vi "Process.vi"(8 "error in":errorcluster, 11 "Instrument UI.FrameworkTemplate":refnum<class "Instrument UI.Temperhum.lvclass">) -> (0 "error out":errorcluster, 3 "Instrument UI.FrameworkTemplate out":refnum<class "Instrument UI.Temperhum.lvclass">)   [LabVIEW 2019, in "Instrument UI.Temperhum.lvclass"]
doc: "---------------------------------------------------------------\nJKI State Machine Objects™\nhttp://jki.net/state-machine-objects/\nCopyright (C) 2005-2015, JKI <info@jki.net>\nALL RIGHTS RESERVEDJKI State Machine Objects (SMO) 1.0.0.5\nJKI - JKI\nCopyright (c) 2016, JKI"
uses:
  Instrument UI.Temperhum.lvclass
  C:/Program Files (x86)/National Instruments/LabVIEW 2019/vi.lib/JKI/JKI SMO/SMO/SMO.lvclass
  C:/Program Files (x86)/National Instruments/LabVIEW 2019/user.lib/LevyLab/Instrument Framework/SMOs/Instrument UI/Instrument UI.lvclass
  C:/Program Files (x86)/National Instruments/LabVIEW 2019/vi.lib/JKI/JKI SMO/SMO.UI/SMO.UI.lvclass
  <vilib>/JKI/JKI SMO/SMO/Typedefs/Parent Call--Enum.ctl
  Instrument.Temperhum/Typedefs/Instrument.Temperhum.getAll--Cluster.ctl
  Instrument.Temperhum/Instrument.Temperhum.lvclass
  C:/Program Files (x86)/National Instruments/LabVIEW 2019/user.lib/LevyLab/Instrument Framework/SMOs/Instrument/Instrument.lvclass
  Instrument UI.Temperhum.UI--Cluster.ctl
  Instrument.Temperhum/Typedefs/Instrument.Temperhum.Configuration--Cluster.ctl
  <userlib>/LevyLab/Instrument Framework/SMOs/Configuration/Configuration.lvclass
  <userlib>/LevyLab/Instrument Framework/SMOs/Instrument UI/Instrument UI.lvclass/Instrument UI.ctl
  Instrument.Temperhum/Instrument.Temperhum.lvclass/Instrument.Temperhum.ctl
  <vilib>/JKI/JKI SMO/SMO/SMO.lvclass/SMO.ctl
  <userlib>/LevyLab/Instrument Framework/SMOs/Instrument/Instrument.lvclass/Instrument.ctl
  614f1787-3484-4d72-b522-1f8c221dac07.vi
  064e3a37-d4cf-416d-9c97-81a00de9d50c.vi
  <vilib>/JKI/JKI SMO/SMO/Private/ReftoDVR--SMO.vi
  614f1787-3484-4d72-b522-1f8c221dac07.vi/0804abc2-d62d-4fc2-83e4-fbfa93b6771f.vi
  064e3a37-d4cf-416d-9c97-81a00de9d50c.vi/63d05343-f2e5-4332-a01c-367bfd4ece1f.vi
  614f1787-3484-4d72-b522-1f8c221dac07.vi/0804abc2-d62d-4fc2-83e4-fbfa93b6771f.vi/49ab1656-e913-41b8-8f65-7ccb5614f4ae.vi
  <userlib>/LevyLab/Instrument Framework/SMOs/Instrument/API/Send and Receive.vi
  <userlib>/LevyLab/Instrument Framework/SMOs/Instrument/API/Read SMO Address.vi
  064e3a37-d4cf-416d-9c97-81a00de9d50c.vi/63d05343-f2e5-4332-a01c-367bfd4ece1f.vi/e8b685cb-2eaa-4147-917d-8853431d5f1e.vi
  614f1787-3484-4d72-b522-1f8c221dac07.vi/0804abc2-d62d-4fc2-83e4-fbfa93b6771f.vi/49ab1656-e913-41b8-8f65-7ccb5614f4ae.vi/5f920abd-0665-4854-95b0-22af96bc7ab8.vi
  614f1787-3484-4d72-b522-1f8c221dac07.vi/0804abc2-d62d-4fc2-83e4-fbfa93b6771f.vi/49ab1656-e913-41b8-8f65-7ccb5614f4ae.vi/ccf45d59-ecb4-4ff7-9932-c5d6b9216eb0.vi
  064e3a37-d4cf-416d-9c97-81a00de9d50c.vi/63d05343-f2e5-4332-a01c-367bfd4ece1f.vi/e8b685cb-2eaa-4147-917d-8853431d5f1e.vi/8176c5a5-7aad-4107-91e7-ec137d50c96d.vi
  064e3a37-d4cf-416d-9c97-81a00de9d50c.vi/63d05343-f2e5-4332-a01c-367bfd4ece1f.vi/e8b685cb-2eaa-4147-917d-8853431d5f1e.vi/514d73de-289c-4ab7-be0e-afcbb581ae6d.vi
  <userlib>/LevyLab/Instrument Framework/SMOs/Instrument/API/Enum to String.vi
  <userlib>/LevyLab/Instrument Framework/SMOs/RemoteControl/API/Send and Receive.vi
  <vilib>/Utility/Data Type/Get Type Information.vi
  <vilib>/JDP Science/JSONtext/JSON text to Variant.vi
  <userlib>/LevyLab/Instrument Framework/SMOs/Instrument/Instrument.lvclass
  <vilib>/JDP Science/JSONtext/LVClass Serializer/JSONtext LVClass Serializer.lvclass
  <userlib>/LevyLab/Instrument Framework/SMOs/Instrument UI/Instrument UI.lvclass
  <vilib>/JKI/JKI SMO/SMO/SMO.lvclass
  <vilib>/JKI/JKI SMO/SMO.UI/SMO.UI.lvclass
  <userlib>/LevyLab/LV-Data/LV-Data.PG/LV-Data.PGSQL.lvclass
panel:
  out "PGSQL":string
  out "TH Graph":cluster{timestamp[], dbl[]}[](graph)
  out "Hardware Type":string
  out "Numeric":u32
  in  "STOP":bool
  out "Humidity (%RH)":dbl
  out "Temperature (K)":dbl
  # "SMO UI Template"
  # "For instructions on how to use the JKI State Machine Objects, examples and video tutorials, visit:\nhttp://jki.net/state-machine-objects/\n\nJKI State Machine Objects™\nhttp://jki.net/state-machine-objects/\nCopyright (C) 2005-2015, JKI <info@jki.net>\nALL RIGHTS RESERVED"
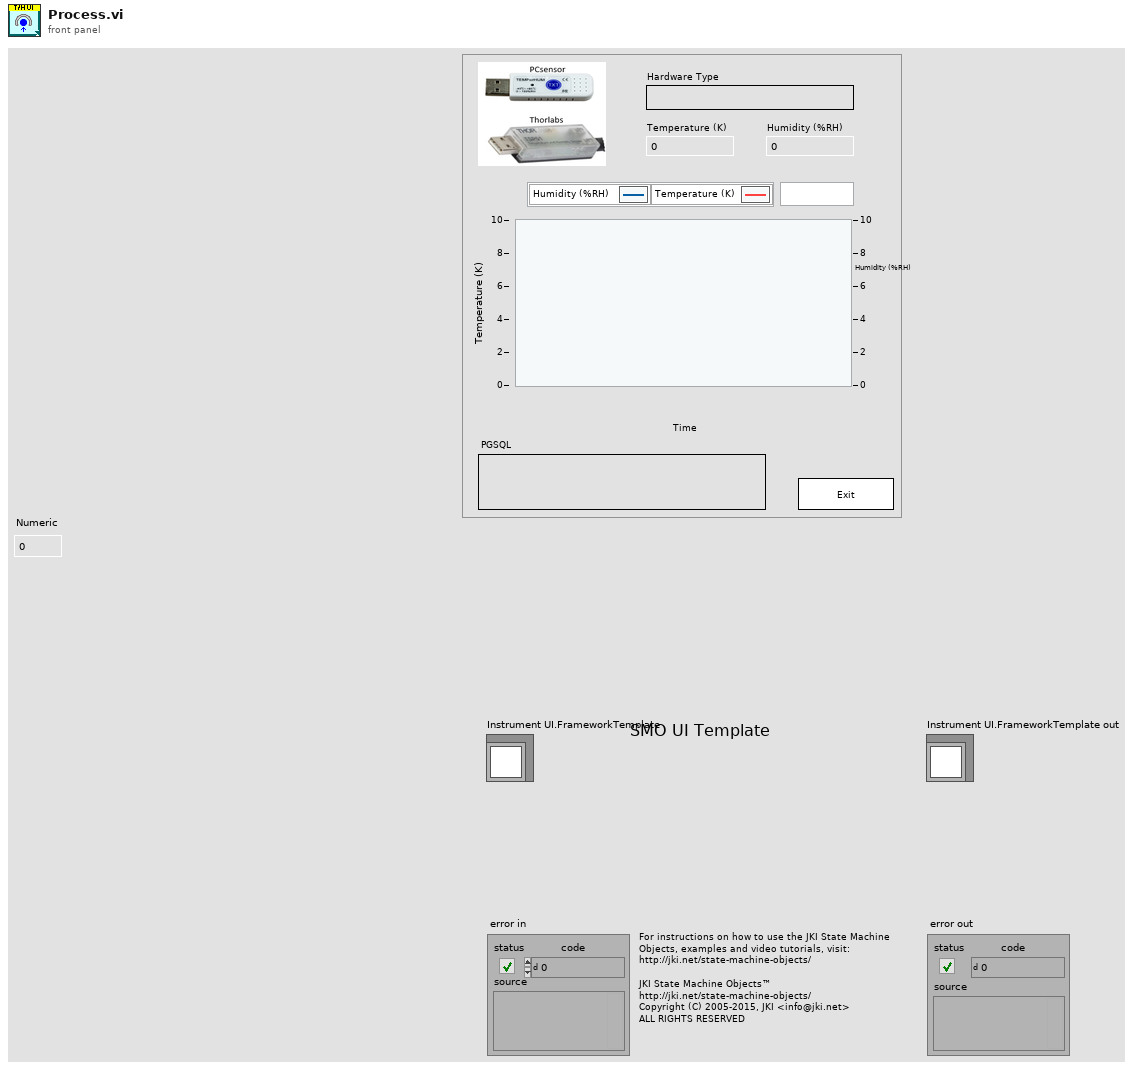
[diagram p1: front panel]
types:
  T1 = typedef "SMO.lvclass/Parent Call--Enum.ctl" = enum16{"Allows parent to run", "Does not request parent to run"}
  T2 = enum32{"invalid app kind", "Development System", "Run Time System", "Student Edition", "Embedded LabVIEW", "Evaluation", "Custom"}
  T3 = enum32{"Invalid", "Standard", "Closed", "Hidden", "Minimized", "Maximized"}
  T4 = typedef "Instrument.Temperhum.lvclass/Instrument.Temperhum.getAll--Cluster.ctl" = cluster{"Temperature (K)":dbl, "Humidity (%RH)":dbl}
  T5 = typedef "Instrument.Temperhum.lvclass/Instrument.Temperhum.Configuration--Cluster.ctl" = cluster{"Example Setting 1":dbl, "Example Setting 2":dbl, "Logpath":string}
  T6 = typedef "Instrument UI.Temperhum.lvclass/Instrument UI.Temperhum.UI--Cluster.ctl" = cluster{"Parameter":dbl, "Parameter 2":string}
  T7 = cluster{"Core":cluster{"Current VI Reference":refnum<vi>, "Close Panel on Exit?":bool, "error":errorcluster}, "Instrument UI":refnum<class "Instrument UI.Temperhum.lvclass">, "Instrument":refnum<class "Instrument.Temperhum.lvclass">, "Configuration":refnum<class "Configuration.lvclass">, "Config Cluster":T5, "getAll":T4, "UI Cluster":T6}
  T8 = typedef "Instrument.Temperhum.lvclass/PublicEvents--Instrument.Temperhum.Get PGSQL Info.ctl" = string
  T9 = cluster{"Current VI Reference":refnum<vi>, "Close Panel on Exit?":bool, "error":errorcluster}
  T10 = typedef "SMO.lvclass/Protected Events.ctl" = cluster{"StopProcesses":refnum<user-event>, "AbortProcesses":refnum<user-event>, "Config Changed":refnum<user-event>, "Dependency":refnum<user-event>}
  T11 = typedef "Instrument.lvclass/PublicEvents--Cluster.ctl" = cluster{"MessageFromProcess":refnum<user-event>}
  T12 = typedef "Instrument.Temperhum.lvclass/PublicEvents--Cluster.ctl" = cluster{"Get PGSQL Info":refnum<user-event>}
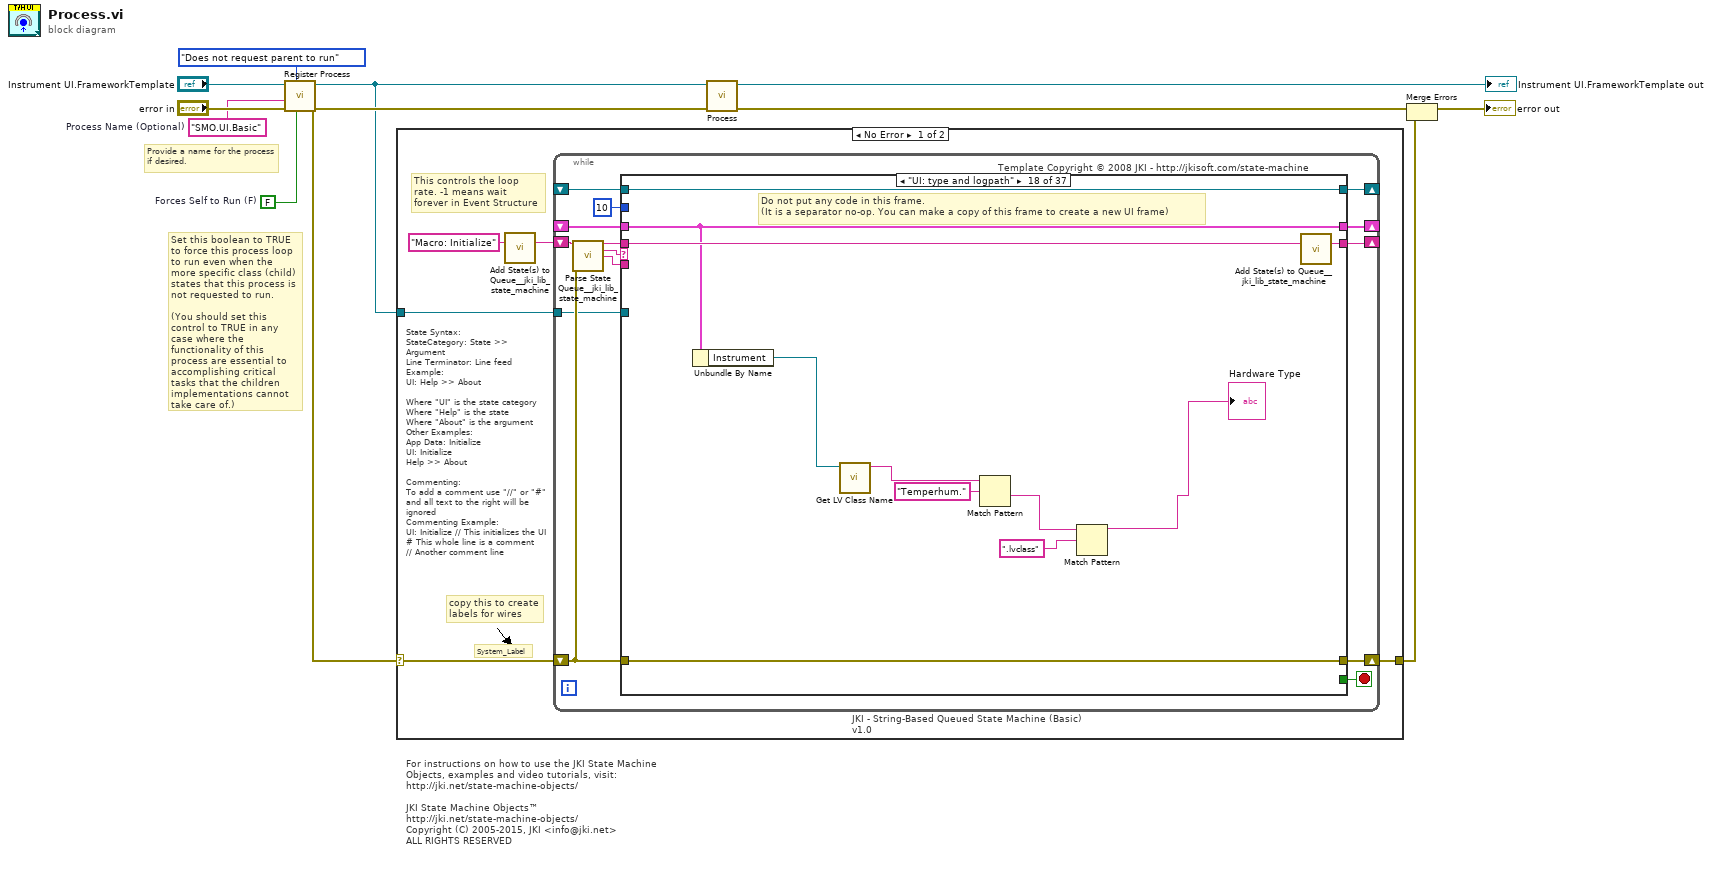
[diagram p0: block diagram]
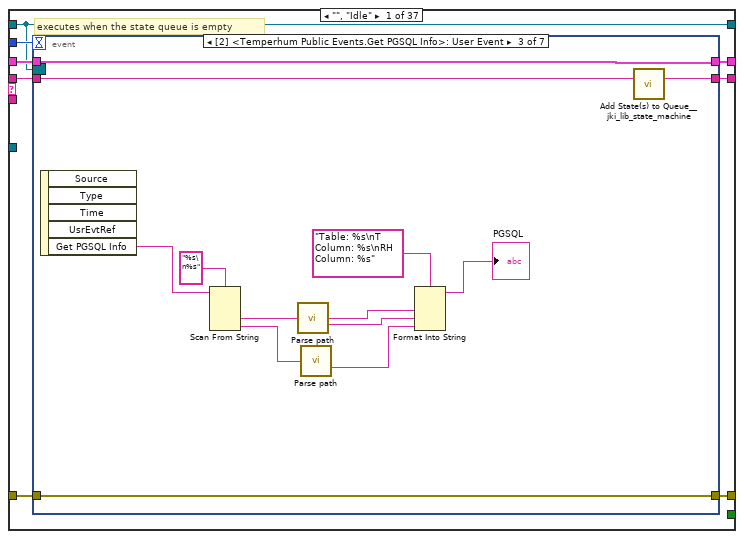
[diagram p2: hidden frame]
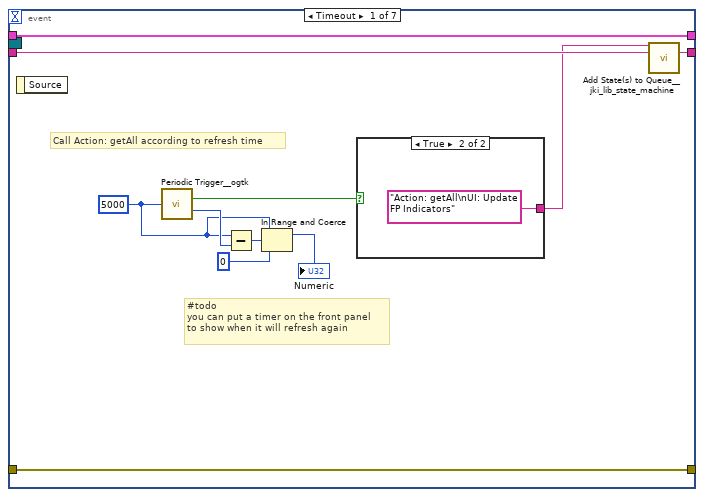
[diagram p3: hidden frame]
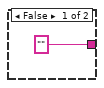
[diagram p4: hidden frame]
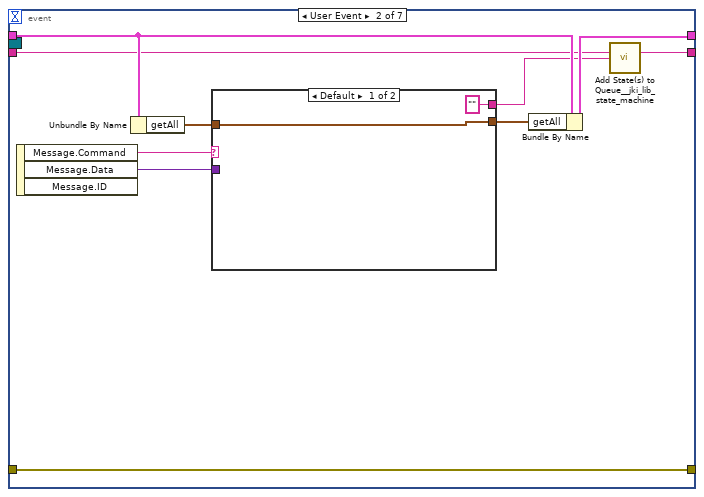
[diagram p5: hidden frame]
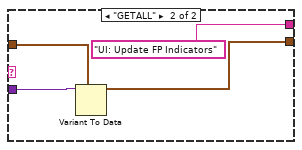
[diagram p6: hidden frame]
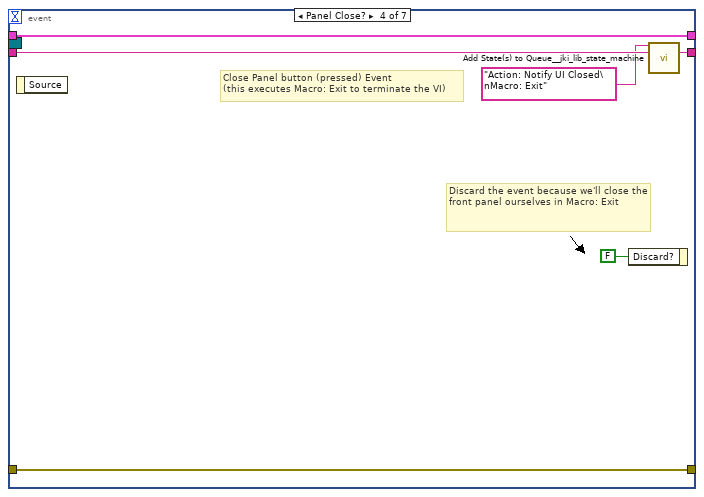
[diagram p7: hidden frame]
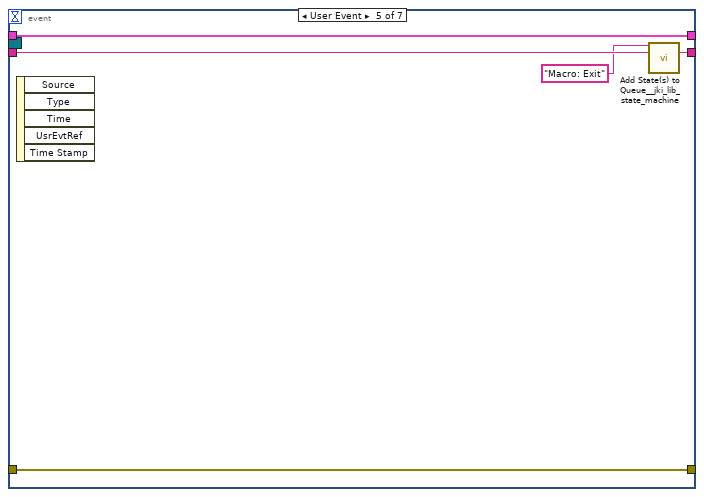
[diagram p8: hidden frame]
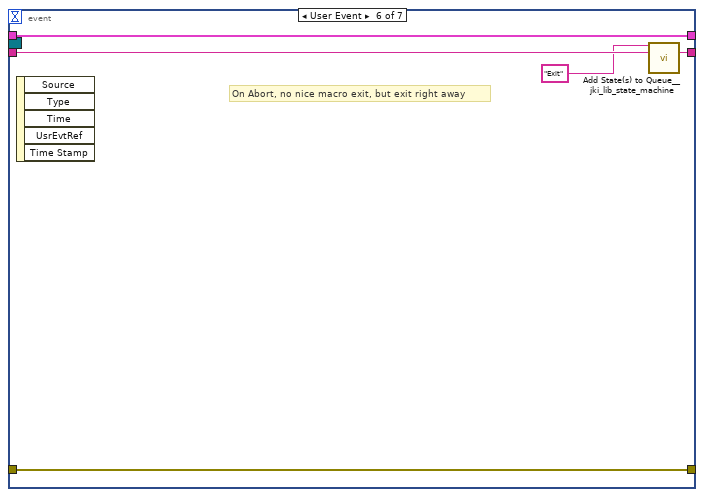
[diagram p9: hidden frame]
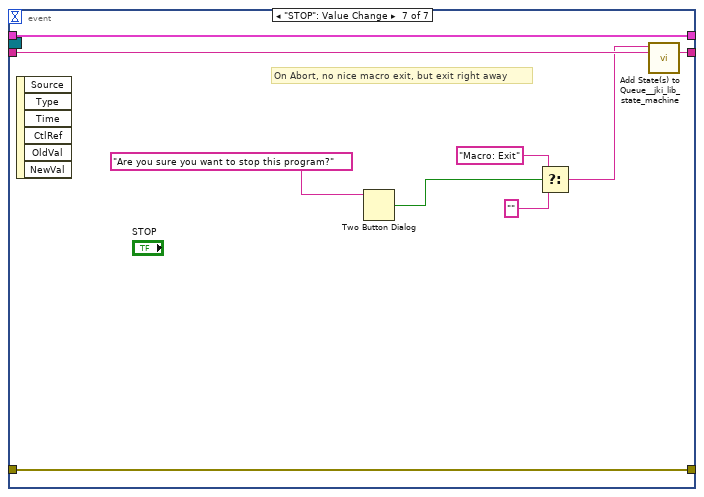
[diagram p10: hidden frame]
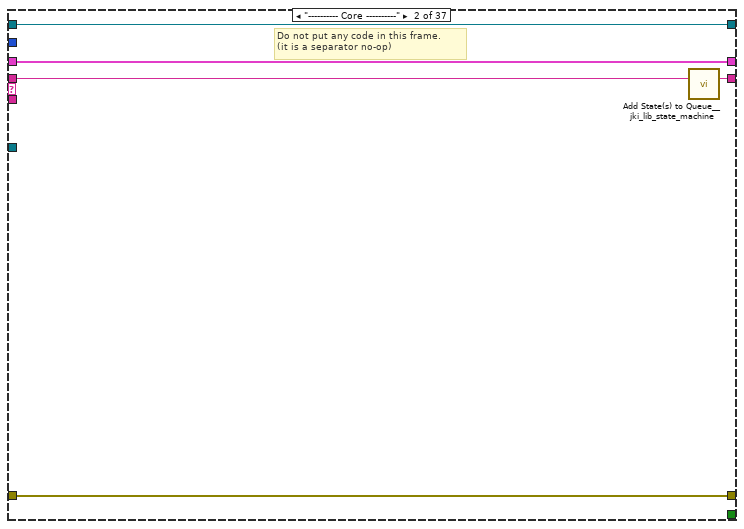
[diagram p11: hidden frame]
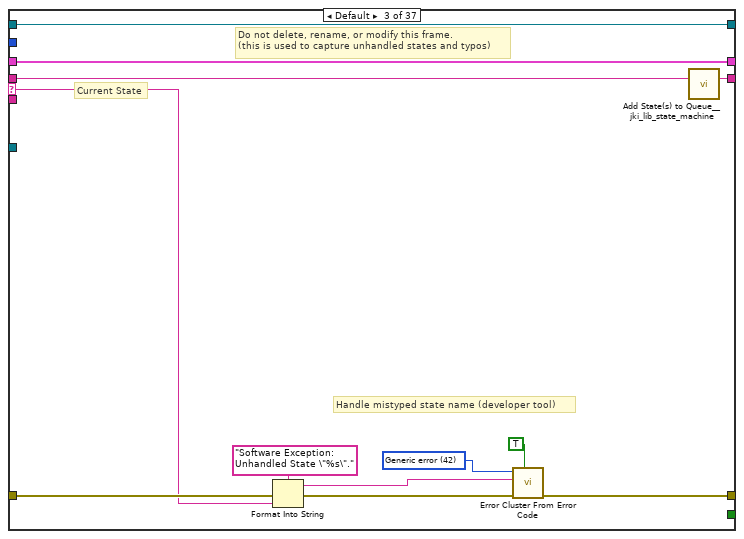
[diagram p12: hidden frame]
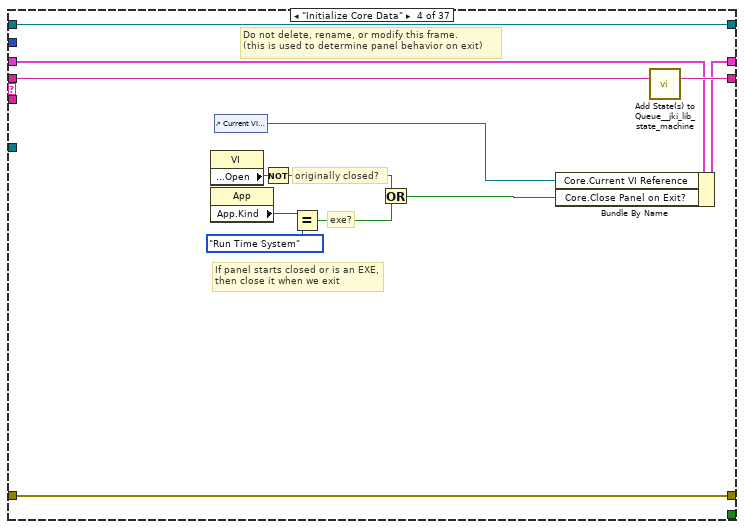
[diagram p13: hidden frame]
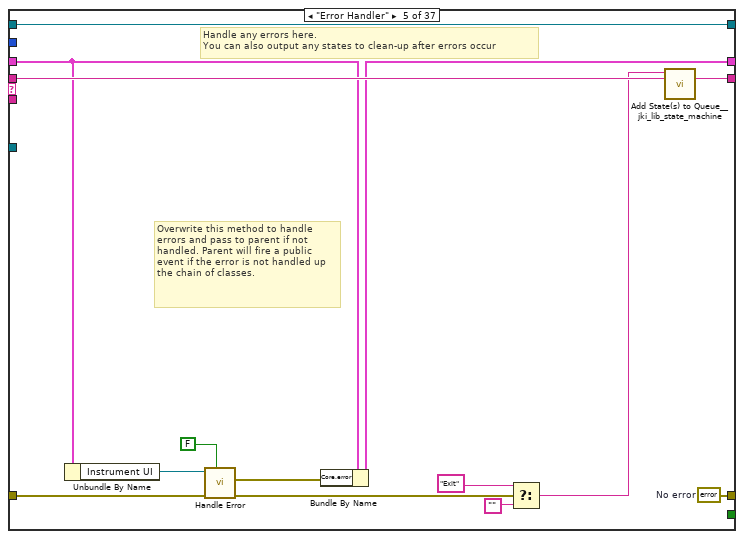
[diagram p14: hidden frame]
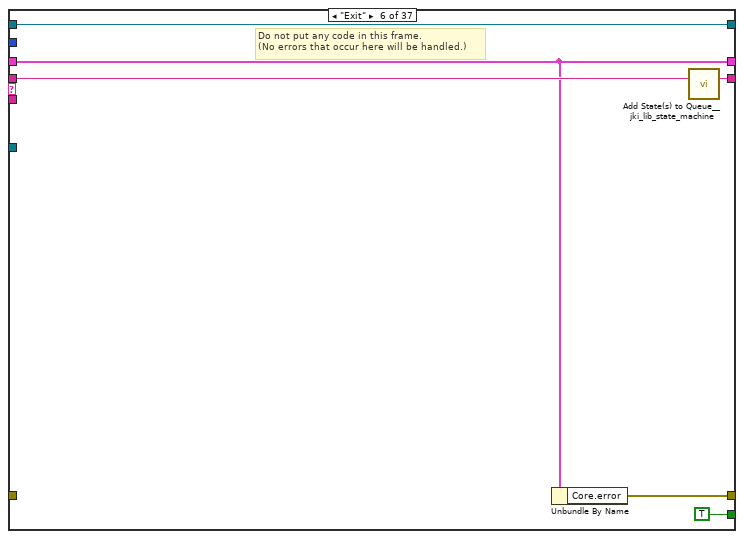
[diagram p15: hidden frame]
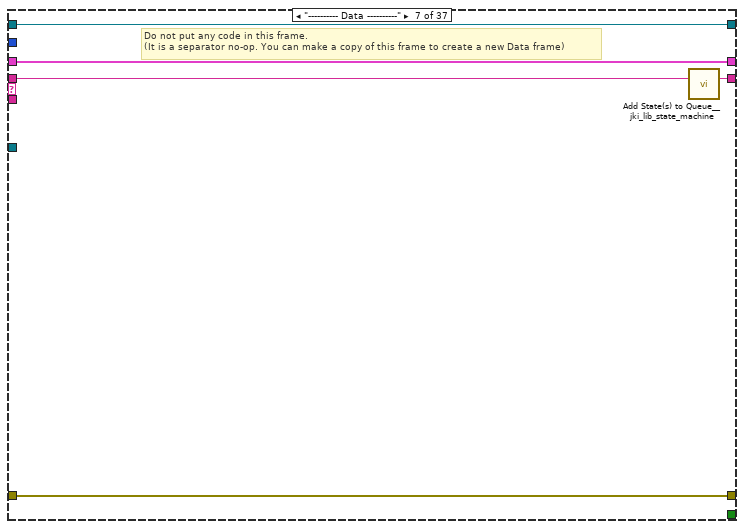
[diagram p16: hidden frame]
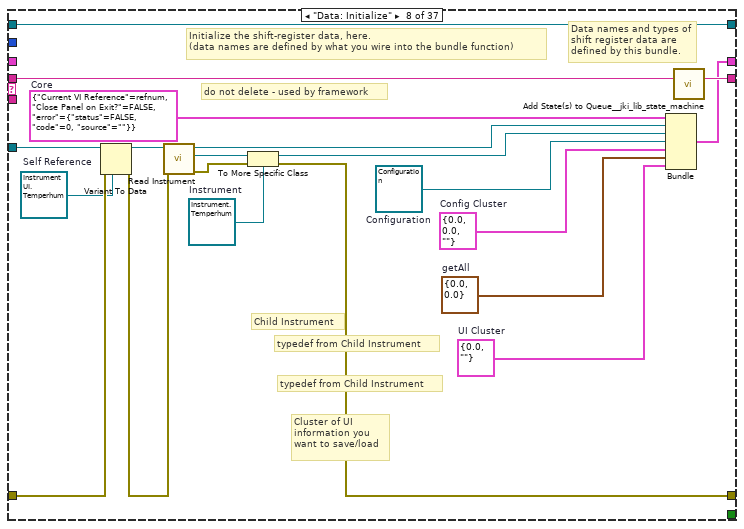
[diagram p17: hidden frame]
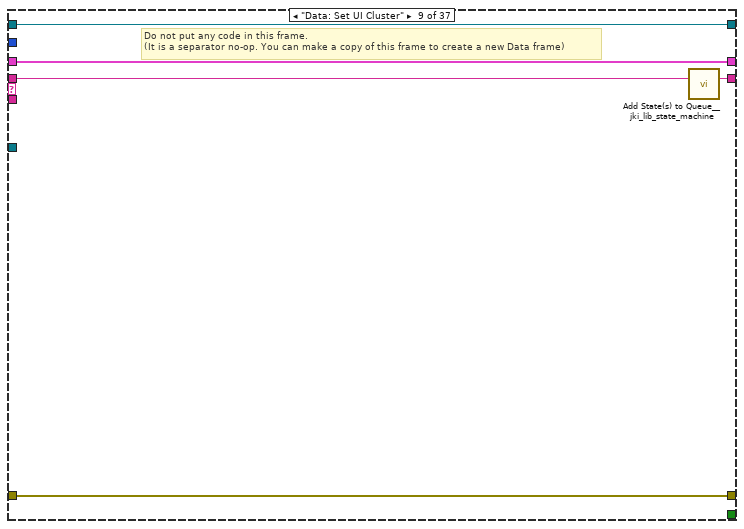
[diagram p18: hidden frame]
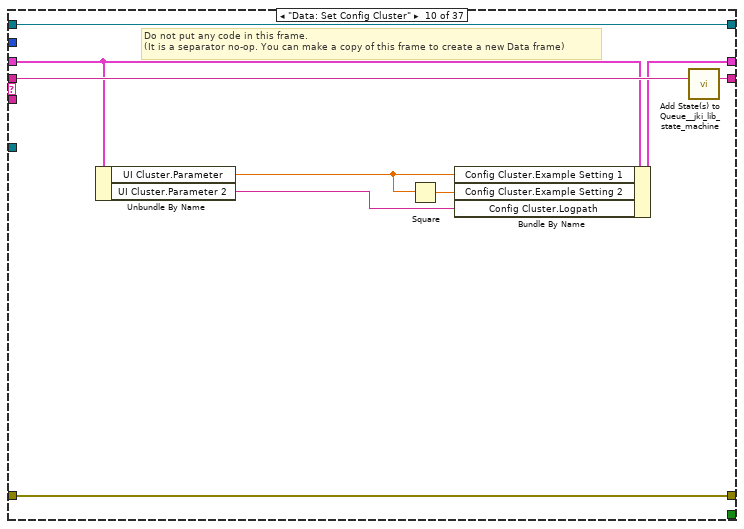
[diagram p19: hidden frame]
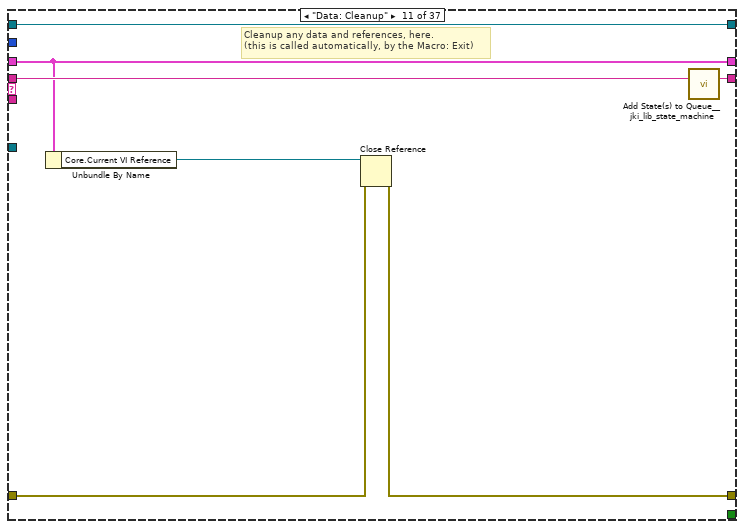
[diagram p20: hidden frame]
diagram:
  w2 = FALSE  # Forces Self to Run (F)
  w1 = "SMO.UI.Basic"  # Process Name (Optional)
  # "Provide a name for the process\nif desired."
  # "Set this boolean to TRUE to force this process loop to run even when the more specific class (child) states that this process is not requested to run.\n\n(You should set this control to TRUE in any case where the functionality of this process are essential to accomplishing critical tasks that the children implementations cannot take care of.)"
  # "For instructions on how to use the JKI State Machine Objects, examples and video tutorials, visit:\nhttp://jki.net/state-machine-objects/\n\nJKI State Machine Objects™\nhttp://jki.net/state-machine-objects/\nCopyright (C) 2005-2015, JKI <info@jki.net>\nALL RIGHTS RESERVED"
  n1 = call <vilib>:"Register Process.vi"("Forces Self to Run (F)"=w2, "Parent Call"=Parent_Call--Enum."Does not request parent to run", "error in (no error)"="error in", "Process Name (optional)"=w1, "SMO"="Instrument UI.FrameworkTemplate") -> ("error out"=w8:errorcluster, "SMO out"=w7:refnum<class "Instrument UI.Temperhum.lvclass">)  [unwired: 5 in]
  n2 = case shown="No Error" w8 {
    selector: w8 -> [w13 w457]
    tunnel: w7 -> [w14 _]
    tunnel: [w12 w457] -> w4
    frame No Error {
      # "State Syntax:\nStateCategory: State >> Argument\nLine Terminator: Line feed\nExample:\nUI: Help >> About\n\nWhere \"UI\" is the state category\nWhere \"Help\" is the state\nWhere \"About\" is the argument\nOther Examples:\nApp Data: Initialize\nUI: Initialize\nHelp >> About\n\nCommenting:\nTo add a comment use \"//\" or \"#\" and all text to the right will be ignored\nCommenting Example:\nUI: Initialize // This initializes the UI\n# This whole line is a comment\n// Another comment line"
      # "copy this to create labels for wires"
      # "This controls the loop rate. -1 means wait forever in Event Structure"
      # "System_Label"
      n3 = call <vilib>:"Add State(s) to Queue__jki_lib_state_machine.vi"("State(s) in (\"\")"="Macro: Initialize") -> ("States Out"=w16:string)  [unwired: 14 in]
      n4 = while "JKI - String-Based Queued State Machine (Basic) v1.0" {
        shift-right: [w23] -> _
        shift-left: _ -> [w22]
        shift-right: [w26] -> w12
        shift-left: w13 -> [w20]
        shift-right: [w25] -> _
        shift-left: w16 -> [w27]
        tunnel: w14 -> [w19]
        shift-right: [w18] -> _
        shift-left: _ -> [w17]
        stop <- w24 stop-if-true
        # "Template Copyright © 2008 JKI - http://jkisoft.com/state-machine"
        n5 = call <vilib>:"Parse State Queue__jki_lib_state_machine.vi"("State Queue"=w27, "Error In (no error)"=w20) -> ("Remaining States"=w29:string, "Current State"=w30:string, "Arguments"=w28:string)  [unwired: 11 in]
        n6 = case shown="\"UI: type and logpath\"" w30 {
          selector: w30 -> [_ _ w112 _ _ _ _ _ _ _ _ _ _ _ _ _ _ _ _ _ _ _ _ _ _ _ _ _ _ _ _ _ _ _ _ _ _]
          tunnel: w29 -> [w38 w110 w116 w135 w149 w155 w160 w180 w185 w194 w201 w206 w214 w219 w230 w237 w253 w291 w296 w305 w311 w317 w332 w337 w348 w355 w360 w376 w382 w387 w399 w407 w419 w426 w433 w445 w456]
          tunnel: w28 -> [_ _ _ _ _ _ _ _ _ _ _ _ _ _ _ w231 w247 _ _ _ _ _ _ _ _ _ _ _ _ _ _ _ _ _ _ _ _]
          tunnel: w22 -> [w36 w107 w114 w126 w138 w151 w157 _ w181 w190 w195 w203 w208 w215 w225 w235 w249 w284 w293 w301 w308 w314 w319 w334 w345 w350 w357 w374 w380 w384 w390 w404 w410 w422 w427 w437 w448]
          tunnel: [w35 w108 w118 w132 w140 w150 w158 w162 w183 w192 w197 w204 w210 w217 w226 w232 w250 w289 w294 w303 w309 w315 w330 w335 w339 w351 w358 w369 w377 w385 w394 w402 w411 w423 w428 w442 w453] -> w26
          tunnel: w20 -> [w34 w108 w117 w132 w145 _ w158 w177 w183 w192 w198 w204 w211 w217 w226 w233 w251 w289 w294 w303 w309 w315 w330 w335 w340 w352 w358 w371 w378 w385 w392 w400 w412 w423 w429 w438 w449]
          tunnel: [w37 w109 w115 w134 w148 w154 w159 w179 w184 w193 w200 w205 w213 w218 w229 w236 w252 w290 w295 w304 w310 w316 w331 w336 w347 w354 w359 w375 w381 w386 w398 w406 w418 w425 w432 w444 w455] -> w25
          tunnel: [_ _ _ _ _ TRUE _ _ _ _ _ _ _ _ _ _ _ _ _ _ _ _ _ _ _ _ _ _ _ _ _ _ _ _ _ _ _] -> w24
          tunnel: [w33 w107 w114 w133 w137 w151 w157 w178 w181 w189 w195 w203 w208 w215 w225 w235 w249 w284 w293 w301 w308 w314 w319 w334 w345 w350 w357 w374 w380 w384 w396 w404 w408 w421 w427 w439 w450] -> w23
          tunnel: 10 ("Timeout") -> [w32 _ _ _ _ _ _ _ _ _ _ _ _ _ _ _ _ _ _ _ _ _ _ _ _ _ _ _ _ _ _ _ _ _ _ _ _]
          tunnel: w19 -> [_ _ _ _ _ _ _ w175 _ _ _ _ _ _ _ _ _ _ _ _ _ _ _ _ _ _ _ _ _ _ _ _ _ _ _ _ _]
          tunnel: [w31 w106 w111 w123 w147 w152 w156 w174 w182 w191 w196 w202 w212 w216 w228 w234 w246 w288 w292 w302 w307 w313 w324 w333 w346 w353 w356 w373 w379 w383 w397 w405 w417 w424 w431 w443 w454] -> w18
          tunnel: w17 -> [w31 w106 w111 w123 w147 w152 w156 w174 w182 w191 w196 w202 w212 w216 w228 w234 w246 w288 w292 w302 w307 w313 w324 w333 w346 w353 w356 _ w379 w383 w397 w405 w417 w424 w431 w443 w454]
          frame "", "Idle" {
            # "executes when the state queue is empty"
            n7 = event shown="[2] <Temperhum Public Events.Get PGSQL Info>: User Event" {
              selector: w31 -> [_ _ _ _ _ _ _]
              dyn-events: _ -> [_ _ _ _ _ _ _]
              timeout: w32 -> [_ _ _ _ _ _ _]
              tunnel: w38 -> [w49 w54 w79 w86 w91 w96 w105]
              tunnel: [w48 w55 w80 w85 w90 w95 w104] -> w37
              tunnel: w36 -> [w46 w56 w77 w82 w88 w93 w102]
              tunnel: [w47 w52 w78 w81 w89 w94 w103] -> w35
              tunnel: w34 -> [w47 w52 w78 w81 w89 w94 w103]
              tunnel: [w46 w57 w77 w82 w88 w93 w102] -> w33
              event Timeout {
                w40 = u32 5000 ("time (ms)")
                # "#todo\nyou can put a timer on the front panel\nto show when it will refresh again"
                # "Call Action: getAll according to refresh time"
                n8 = event-data() -> ()  [unwired: 1 in, 1 out]
                n9 = call <userlib>:"Periodic Trigger__ogtk.vi"("time (ms)"=w40) -> ("Triggered"=w44:bool, "timer value"=w43:u32)  [unwired: 12 in, 1 out]
                n10 = Subtract(x=w40, y=w43) -> (x-y=w42:u32)
                n11 = In Range and Coerce(upper limit=w40, x=w42, lower limit=u32 0) -> (coerced(x)=→"Numeric":u32)  [unwired: 1 out]
                n12 = case shown="True" w44 {
                  tunnel: ["" ("State(s) in Front (\"\")") "Action: getAll\nUI: Update FP Indicators" ("State(s) in Front (\"\")")] -> w45
                  frame False {
                  }
                  frame True {
                  }
                }
                n13 = call <vilib>:"Add State(s) to Queue__jki_lib_state_machine.vi"("State(s) in Front (\"\")"=w45, "State(s) in (\"\")"=w49) -> ("States Out"=w48:string)  [unwired: 13 in]
              }
              event User Event {
                n14 = event-data() -> ("Message.Command"=w61:string, "Message.Data"=w60:variant)  [unwired: 1 in, 1 out]
                n15 = Unbundle By Name(w56) -> ("getAll"=w59:T4)
                n16 = case shown="Default" w61 {
                  tunnel: w60 -> [_ w67]
                  tunnel: w59 -> [w63 w66]
                  tunnel: [w63 w65] -> w58
                  tunnel: ["" "UI: Update FP Indicators"] -> w53
                  frame Default {
                  }
                  frame "GETALL" {
                    n17 = Variant To Data(type=w66, Variant=w67) -> (data=w65:T4)  [unwired: 1 in, 1 out]
                  }
                }
                n18 = Bundle By Name(cluster=w56, "getAll"=w58) -> (w57:T7)
                n19 = call <vilib>:"Add State(s) to Queue__jki_lib_state_machine.vi"("State(s) in (\"\")"=w54, "State(s) at Back (\"\")"=w53) -> ("States Out"=w55:string)  [unwired: 13 in]
              }
              event User Event {
                n20 = event-data() -> ("Get PGSQL Info"=w76:T8)  [unwired: 1 in, 4 out]
                n21 = Scan From String(format string="%s\n%s", input string=w76) -> (output 1=w74:string, output 2=w73:string)  [unwired: 4 in, 3 out]
                n22 = call <userlib>:"Parse path.vi"("PG Path"=w74) -> ("Table name"=w70:string, "Column name"=w69:string)  [unwired: 10 in, 3 out]
                n23 = call <userlib>:"Parse path.vi"("PG Path"=w73) -> ("Column name"=w68:string)  [unwired: 10 in, 4 out]
                n24 = Format Into String(format string="Table: %s\nT Column: %s\nRH Column: %s", w70, w69, w68) -> (resulting string=→"PGSQL":string)  [unwired: 2 in, 1 out]
                n25 = call <vilib>:"Add State(s) to Queue__jki_lib_state_machine.vi"("State(s) in (\"\")"=w79) -> ("States Out"=w80:string)  [unwired: 14 in]
              }
              event Panel Close? {
                # "Discard the event because we'll close the front panel ourselves in Macro: Exit"
                # "Close Panel button (pressed) Event\n(this executes Macro: Exit to terminate the VI)"
                n26 = event-data() -> ()  [unwired: 1 in, 1 out]
                n27 = event-data("Discard?"=FALSE) -> ()  [unwired: 1 in, 1 out]
                n28 = call <vilib>:"Add State(s) to Queue__jki_lib_state_machine.vi"("State(s) in Front (\"\")"="Action: Notify UI Closed\nMacro: Exit", "State(s) in (\"\")"=w86) -> ("States Out"=w85:string)  [unwired: 13 in]
              }
              event User Event {
                n29 = event-data() -> ()  [unwired: 1 in, 5 out]
                n30 = call <vilib>:"Add State(s) to Queue__jki_lib_state_machine.vi"("State(s) in Front (\"\")"="Macro: Exit", "State(s) in (\"\")"=w91) -> ("States Out"=w90:string)  [unwired: 13 in]
              }
              event User Event {
                # "On Abort, no nice macro exit, but exit right away"
                n31 = event-data() -> ()  [unwired: 1 in, 5 out]
                n32 = call <vilib>:"Add State(s) to Queue__jki_lib_state_machine.vi"("State(s) in Front (\"\")"="Exit", "State(s) in (\"\")"=w96) -> ("States Out"=w95:string)  [unwired: 13 in]
              }
              event "STOP": Value Change {
                # "On Abort, no nice macro exit, but exit right away"
                n33 = event-data() -> ()  [unwired: 1 in, 6 out]
                n34 = Two Button Dialog(message="Are you sure you want to stop this program?") -> (T button?=w101:bool)  [unwired: 2 in]
                n35 = Select(t="Macro: Exit", s=w101, f="") -> (s? t:f=w97:string)
                n36 = call <vilib>:"Add State(s) to Queue__jki_lib_state_machine.vi"("State(s) in Front (\"\")"=w97, "State(s) in (\"\")"=w105) -> ("States Out"=w104:string)  [unwired: 13 in]
              }
            }
          }
          frame "---------- Core ----------" {
            # "Do not put any code in this frame.\n(it is a separator no-op)"
            n37 = call <vilib>:"Add State(s) to Queue__jki_lib_state_machine.vi"("State(s) in (\"\")"=w110) -> ("States Out"=w109:string)  [unwired: 14 in]
          }
          frame Default {
            w121 = 42 items=["No error", "Argument error", "Memory is full", "Out of zone", "End of file", "File already open", "Generic file I/O error", "File not found", "File permission error", "Disk is full", "Duplicate path", "Too many files open", "System feature not enabled", "Resource file not found", "Cannot add resource", "Resource not found", "Image not found", "Image memory error", "Pen does not exist", "Config type invalid", "Config token not found", "Config parse error", "Config memory error", "Bad external code format", "Bad external code offset", "External code not present", "Null window", "Destroy window error", "Null menu", "Print aborted", "Bad print record", "Print driver error", "Windows error during printing", "Memory error during printing", "Print dialog error", "Generic print error", "Invalid device refnum", "Device not found", "Device parameter error", "Device unit error", "Cannot open device", "Device call aborted", "Generic error", "Cancelled by user", "Object ID too low", "Object ID too high", "Object not in heap", "Unknown heap", "Unknown object (invalid DefProc)", "Unknown object (DefProc not in table)", "Message out of range", "Invalid (null) method", "Unknown message", "Manager call not supported", "Bad address", "Network operation in progress", "Network operation timed out", "Connection is busy", "Network attribute not supported", "Network error", "Address in use", "System out of memory", "Connection aborted", "Connection refused", "Not connected", "Already connected", "Connection closed", "Initialization error (interapplication manager)", "Bad occurrence", "Wait on unbound occurrence handler", "Occurrence queue overflow", "Datalog type conflict", "Unused", "Unrecognized type (interapplication manager)", "Memory corrupt", "Failed to make temporary DLL", "Old CIN version", "Drag socket not found", "Failed to load drop-object", "Failed to register OLE object", "Failed to release OLE object", "Format specifier type mismatch", "Unknown format specifier", "Too few format specifiers", "Too many format specifiers", "Scan failed", "Newer CIN version", "Error converting to variant", "Runtime menu error", "Password tampered", "Variant attribute not found", "Incompatible variant data type", "Event data is not available", "Event Store is not present", "Occurrence is not found", "Event Queue is not created", "Event info is not available", "Refnum passed is NULL", "Error retrieving Class GUID", "Error retrieving CoClass GUID", "Error retrieving TypeLib GUID.", "Bad built application magic bytes.", "Specific driver is different from the specific driver associated with the Logical Name.", "There is no session opened to the class driver.", "Max Error", "MAX - Error with config objects", "MAX - Error loading configuration", "MAX - Group not supported"]
            # "Current State"
            # "Do not delete, rename, or modify this frame.\n(this is used to capture unhandled states and typos)"
            # "Handle mistyped state name (developer tool)"
            n38 = Format Into String(format string="Software Exception: Unhandled State \"%s\"." ("message"), error in=w117, w112) -> (resulting string=w120:string, error out=w119:errorcluster)  [unwired: 1 in]
            n39 = call <vilib>:"Error Cluster From Error Code.vi"("show call chain? (False)"=TRUE, "error in (no error)"=w119, "error message (\"\")"=w120, "error code (0)"=w121) -> ("error out"=w118:errorcluster)  [unwired: 5 in]
            n40 = call <vilib>:"Add State(s) to Queue__jki_lib_state_machine.vi"("State(s) in (\"\")"=w116) -> ("States Out"=w115:string)  [unwired: 14 in]
          }
          frame "Initialize Core Data" {
            # "Do not delete, rename, or modify this frame.\n(this is used to determine panel behavior on exit)"
            # "originally closed?"
            # "exe?"
            # "If panel starts closed or is an EXE, then close it when we exit"
            n41 = property class="VI"() -> ("Front Panel.Open"=w131:bool)  [unwired: 2 in, 2 out]
            n42 = property class="App"() -> ("App.Kind"=w130:T2)  [unwired: 2 in, 2 out]
            n43 = control-ref of="Current VI Reference"() -> (w124:refnum<vi>)
            n44 = Not(x=w131) -> (.not. x?=w128:bool)
            n45 = Equal?(x=w130, y=T2."Run Time System" ("Application:Kind")) -> (x = y?=w127:bool)
            n46 = Or(x=w128, y=w127) -> (x .or. y?=w125:bool)
            n47 = Bundle By Name(cluster=w126, "Core.Current VI Reference"=w124, "Core.Close Panel on Exit?"=w125) -> (w133:T7)
            n48 = call <vilib>:"Add State(s) to Queue__jki_lib_state_machine.vi"("State(s) in (\"\")"=w135) -> ("States Out"=w134:string)  [unwired: 14 in]
          }
          frame "Error Handler" {
            w140 = errorcluster {"status"=FALSE, "code"=0, "source"=""}  # No error
            # "Overwrite this method to handle errors and pass to parent if not handled. Parent will fire a public event if the error is not handled up the chain of classes."
            # "Handle any errors here.\nYou can also output any states to clean-up after errors occur"
            n49 = Unbundle By Name(w138) -> ("Instrument UI"=w146:refnum<class "Instrument UI.Temperhum.lvclass">)
            n50 = call-dynamic "Handle Error.vi"("Stop on Unhandled Error (T)"=FALSE, "error in"=w145, "SMO"=w146) -> ("handling error"=w141:errorcluster, "Unhandled error"=w139:errorcluster)  [unwired: 6 in, 1 out]
            n51 = Bundle By Name(cluster=w138, "Core.error"=w139) -> (w137:T7)
            n52 = Select(t="Exit", s=w141, f="") -> (s? t:f=w142:string)
            n53 = call <vilib>:"Add State(s) to Queue__jki_lib_state_machine.vi"("State(s) in Front (\"\")"=w142, "State(s) in (\"\")"=w149) -> ("States Out"=w148:string)  [unwired: 13 in]
          }
          frame "Exit" {
            # "Do not put any code in this frame.\n(No errors that occur here will be handled.)"
            n54 = Unbundle By Name(w151) -> ("Core.error"=w150:errorcluster)
            n55 = call <vilib>:"Add State(s) to Queue__jki_lib_state_machine.vi"("State(s) in (\"\")"=w155) -> ("States Out"=w154:string)  [unwired: 14 in]
          }
          frame "---------- Data ----------" {
            # "Do not put any code in this frame.\n(It is a separator no-op. You can make a copy of this frame to create a new Data frame)"
            n56 = call <vilib>:"Add State(s) to Queue__jki_lib_state_machine.vi"("State(s) in (\"\")"=w160) -> ("States Out"=w159:string)  [unwired: 14 in]
          }
          frame "Data: Initialize" {
            w161 = refnum<class "Configuration.lvclass"> refnum  # Configuration
            w164 = T5 {"Example Setting 1"=0.0, "Example Setting 2"=0.0, "Logpath"=""}  # Config Cluster
            w166 = T6 {"Parameter"=0.0, "Parameter 2"=""}  # UI Cluster
            w168 = refnum<class "Instrument.Temperhum.lvclass"> refnum  # Instrument
            w172 = T4 {"Temperature (K)"=0.0, "Humidity (%RH)"=0.0}  # getAll
            w173 = T9 {"Current VI Reference"=refnum, "Close Panel on Exit?"=FALSE, "error"={"status"=FALSE, "code"=0, "source"=""}}  # Core
            w176 = refnum<class "Instrument UI.Temperhum.lvclass"> refnum  # Self Reference
            # "typedef from Child Instrument"
            # "Cluster of UI\ninformation you\nwant to save/load"
            # "Child Instrument"
            # "typedef from Child Instrument"
            # "do not delete - used by framework"
            # "Data names and types of shift register data are defined by this bundle."
            # "Initialize the shift-register data, here.\n(data names are defined by what you wire into the bundle function)"
            n57 = Variant To Data(error in=w177, type=w176, Variant=w175) -> (data=w170:refnum<class "Instrument UI.Temperhum.lvclass">, error out=w171:errorcluster)
            n58 = call <userlib>:"Read Instrument.vi"("error in (no error)"=w171, "Instrument UI in"=w170) -> ("error out"=w165:errorcluster, "Instrument"=w167:refnum<class "Instrument.lvclass">, "Instrument UI"=w169:refnum<class "Instrument UI.Temperhum.lvclass">)  [unwired: 7 in]
            n59 = To More Specific Class(target class=w168, reference=w167, error in=w165) -> (specific class reference=w163:refnum<class "Instrument.Temperhum.lvclass">, error out=w162:errorcluster)
            n60 = Bundle("Core"=w173, "Instrument UI"=w169, "Instrument"=w163, "Configuration"=w161, "Config Cluster"=w164, "getAll"=w172, "UI Cluster"=w166) -> (w178:T7)  [unwired: 1 in]
            n61 = call <vilib>:"Add State(s) to Queue__jki_lib_state_machine.vi"("State(s) in (\"\")"=w180) -> ("States Out"=w179:string)  [unwired: 14 in]
          }
          frame "Data: Set UI Cluster" {
            # "Do not put any code in this frame.\n(It is a separator no-op. You can make a copy of this frame to create a new Data frame)"
            n62 = call <vilib>:"Add State(s) to Queue__jki_lib_state_machine.vi"("State(s) in (\"\")"=w185) -> ("States Out"=w184:string)  [unwired: 14 in]
          }
          frame "Data: Set Config Cluster" {
            # "Do not put any code in this frame.\n(It is a separator no-op. You can make a copy of this frame to create a new Data frame)"
            n63 = Unbundle By Name(w190) -> ("UI Cluster.Parameter"=w187:dbl, "UI Cluster.Parameter 2"=w188:string)
            n64 = Square(x=w187) -> (x^2=w186:dbl)
            n65 = Bundle By Name(cluster=w190, "Config Cluster.Example Setting 1"=w187, "Config Cluster.Example Setting 2"=w186, "Config Cluster.Logpath"=w188) -> (w189:T7)
            n66 = call <vilib>:"Add State(s) to Queue__jki_lib_state_machine.vi"("State(s) in (\"\")"=w194) -> ("States Out"=w193:string)  [unwired: 14 in]
          }
          frame "Data: Cleanup" {
            # "Cleanup any data and references, here.\n(this is called automatically, by the Macro: Exit)"
            n67 = Unbundle By Name(w195) -> ("Core.Current VI Reference"=w199:refnum<vi>)
            n68 = Close Reference(reference=w199, error in (no error)=w198) -> (error out=w197:errorcluster)
            n69 = call <vilib>:"Add State(s) to Queue__jki_lib_state_machine.vi"("State(s) in (\"\")"=w201) -> ("States Out"=w200:string)  [unwired: 14 in]
          }
          frame "---------- UI ----------" {
            # "Do not put any code in this frame.\n(It is a separator no-op. You can make a copy of this frame to create a new UI frame)"
            n70 = call <vilib>:"Add State(s) to Queue__jki_lib_state_machine.vi"("State(s) in (\"\")"=w206) -> ("States Out"=w205:string)  [unwired: 14 in]
          }
          frame "UI: Initialize" {
            # "size window to decoration box on front panel"
            # "Initialize the User Interface, here.\n(this is called automatically, by the Macro: Init)"
            n71 = invoke on="STOP" class="Bool (strict)" method="Reinit To Default"() -> ()  [unwired: 3 in, 3 out]
            n72 = call <userlib>:"Fit VI window to Largest Dec__ogtk.vi"("error in (no error)"=w211, "border spacing (2 px)"=0) -> ("error out"=w210:errorcluster)  [unwired: 4 in, 1 out]
            n73 = call <vilib>:"Add State(s) to Queue__jki_lib_state_machine.vi"("State(s) in (\"\")"=w214, "State(s) at Back (\"\")"="UI: type and logpath" ("State(s) at Back (\"\")")) -> ("States Out"=w213:string)  [unwired: 13 in]
          }
          frame "UI: Update FP Controls" {
            # "Do not put any code in this frame.\n(It is a separator no-op. You can make a copy of this frame to create a new UI frame)"
            n74 = call <vilib>:"Add State(s) to Queue__jki_lib_state_machine.vi"("State(s) in (\"\")"=w219) -> ("States Out"=w218:string)  [unwired: 14 in]
          }
          frame "UI: Update FP Indicators" {
            # "do this way to have nicer UI or only display what you want"
            n75 = Unbundle By Name(w225) -> ("getAll"=w227:T4)
            n76 = Unbundle By Name(w227) -> ("Temperature (K)"=w220:dbl, "Humidity (%RH)"=w221:dbl)
            "Temperature (K)" <- w220
            "Humidity (%RH)" <- w221
            n77 = Build Array(w221, w220) -> (w223:dbl[])
            n78 = local read "TH Graph"() -> (w222:cluster{timestamp[], dbl[]}[])
            n79 = call "Time-Y Circ Buffer.vi"("Y in"=w223, "XY in"=w222) -> ("XY"=→"TH Graph":cluster{timestamp[], dbl[]}[])  [unwired: 9 in]
            n80 = call <vilib>:"Add State(s) to Queue__jki_lib_state_machine.vi"("State(s) in (\"\")"=w230) -> ("States Out"=w229:string)  [unwired: 14 in]
          }
          frame "UI: Cursor Set" {
            # "Argument"
            # "Initialize the User Interface, here.\n(this is called automatically, by the Macro: Init)"
            n81 = disable-structure shown="Default" {
              disable-tunnel: w233 -> [w238 w241]
              disable-tunnel: [w238 w240] -> w232
              disable-tunnel: w231 -> [_ w239]
              frame condition #0 {
              }
              frame condition #1 (active) {
                n82 = case shown="\"Busy\"" w239 {
                  tunnel: w241 -> [w243 w245]
                  tunnel: [w242 w244] -> w240
                  frame "Idle", Default {
                    n83 = call <vilib>:"Unset Busy.vi"("error in (no error)"=w243) -> ("error out"=w242:errorcluster)  [unwired: 10 in]
                  }
                  frame "Busy" {
                    n84 = call <vilib>:"Set Busy.vi"("error in (no error)"=w245) -> ("error out"=w244:errorcluster)  [unwired: 9 in, 1 out]
                  }
                }
              }
            }
            n85 = call <vilib>:"Add State(s) to Queue__jki_lib_state_machine.vi"("State(s) in (\"\")"=w237) -> ("States Out"=w236:string)  [unwired: 14 in]
          }
          frame "UI: Front Panel State" {
            # "Argument"
            # "Set Front Panel Open or Closed\n(Usage: \"UI: Front Panel State >> Open|Close\")"
            n86 = Unbundle By Name(w249) -> ("Core.Current VI Reference"=w248:refnum<vi>)
            n87 = disable-structure shown="Default" {
              disable-tunnel: w251 -> [w257 w280]
              disable-tunnel: [w256 w280] -> w250
              disable-tunnel: w248 -> [w255 _]
              disable-tunnel: w247 -> [w254 _]
              frame condition #0 (active) {
                n88 = case shown="\"Close\"" w254 {
                  tunnel: w257 -> [w261 w274]
                  tunnel: [w263 w275] -> w256
                  tunnel: w255 -> [w262 w272]
                  frame "Open", Default {
                    n89 = property class="VI"(reference=w262, error in=w261) -> (reference out=w259:refnum<vi>, error out=w260:errorcluster, "FP.State"=w258:T3)
                    n90 = case shown="\"Closed\"" w258 {
                      tunnel: [w266 w269] -> w263
                      tunnel: w260 -> [w265 w269]
                      tunnel: w259 -> [w264 _]
                      frame "Closed" {
                        n91 = invoke class="VI" method="FP.Open"(reference=w264, error in=w265, "Activate"=TRUE, "State"=T3."Standard") -> (error out=w266:errorcluster)  [unwired: 1 in, 4 out]
                      }
                      frame Default {
                      }
                    }
                  }
                  frame "Close" {
                    n92 = property class="VI"(reference=w272, error in=w274) -> (reference out=w271:refnum<vi>, error out=w273:errorcluster, "FP.State"=w270:T3)
                    n93 = case shown="Default" w270 {
                      tunnel: [w276 w279] -> w275
                      tunnel: w273 -> [w276 w278]
                      tunnel: w271 -> [_ w277]
                      frame "Invalid", "Closed" {
                      }
                      frame Default {
                        n94 = invoke class="VI" method="FP.Close"(reference=w277, error in=w278) -> (error out=w279:errorcluster)  [unwired: 1 in, 2 out]
                      }
                    }
                  }
                }
              }
              frame condition #1 {
              }
            }
            n95 = call <vilib>:"Add State(s) to Queue__jki_lib_state_machine.vi"("State(s) in (\"\")"=w253) -> ("States Out"=w252:string)  [unwired: 14 in]
          }
          frame "UI: type and logpath" {
            # "Do not put any code in this frame.\n(It is a separator no-op. You can make a copy of this frame to create a new UI frame)"
            n96 = Unbundle By Name(w284) -> ("Instrument"=w285:refnum<class "Instrument.Temperhum.lvclass">)
            n97 = call <vilib>:"Get LV Class Name.vi"("object"=w285) -> ("class name"=w287:string)  [unwired: 9 in, 1 out]
            n98 = Match Pattern(string=w287, regular expression="Temperhum.") -> (after substring=w282:string)  [unwired: 1 in, 3 out]
            n99 = Match Pattern(string=w282, regular expression=".lvclass") -> (before substring=→"Hardware Type":string)  [unwired: 1 in, 3 out]
            n100 = call <vilib>:"Add State(s) to Queue__jki_lib_state_machine.vi"("State(s) in (\"\")"=w291) -> ("States Out"=w290:string)  [unwired: 14 in]
          }
          frame "---------- Macro ----------" {
            # "Do not put any code in this frame.\n(It is a separator no-op. You can make a copy of this frame to create a new Macro frame)"
            n101 = call <vilib>:"Add State(s) to Queue__jki_lib_state_machine.vi"("State(s) in (\"\")"=w296) -> ("States Out"=w295:string)  [unwired: 14 in]
          }
          frame "Macro: Initialize" {
            w299 = "UI: Initialize\nMacro: Read UI Config\n//UI: Front Panel State >> Open"  # UI: Initialize Macro: Read UI Config //UI: Front Panel State >> Open
            # "Initialization Macro\n(This is called once, when the VI starts)"
            n102 = call <vilib>:"Add State(s) to Queue__jki_lib_state_machine.vi"("State(s) in Front (\"\")"="Data: Initialize\nInitialize Core Data\nEvents: Register", "State(s) in (\"\")"="Process: Sync", "State(s) at Back (\"\")"=w299) -> ("States Out"=w298:string)  [unwired: 12 in]
            n103 = call <vilib>:"Add State(s) to Queue__jki_lib_state_machine.vi"("State(s) in Front (\"\")"=w298, "State(s) in (\"\")"=w305) -> ("States Out"=w304:string)  [unwired: 13 in]
          }
          frame "Macro: Read UI Config" {
            # "Do not put any code in this frame.\n(It is a separator no-op. You can make a copy of this frame to create a new Macro frame)"
            n104 = call <vilib>:"Add State(s) to Queue__jki_lib_state_machine.vi"("State(s) in Front (\"\")"="Configuration: Initialize\nConfiguration: Read UI Config File\nUI: Update FP Controls" ("State(s) in Front (\"\")"), "State(s) in (\"\")"=w311) -> ("States Out"=w310:string)  [unwired: 13 in]
          }
          frame "Macro: Write UI Config" {
            # "Do not put any code in this frame.\n(It is a separator no-op. You can make a copy of this frame to create a new Macro frame)"
            n105 = call <vilib>:"Add State(s) to Queue__jki_lib_state_machine.vi"("State(s) in Front (\"\")"="Data: Set UI Cluster\nConfiguration: Write UI Config File" ("State(s) in Front (\"\")"), "State(s) in (\"\")"=w317) -> ("States Out"=w316:string)  [unwired: 13 in]
          }
          frame "Macro: Exit" {
            # "Exit Macro\n(This is called once, when the VI exits)"
            n106 = Unbundle By Name(w319) -> ("Core.Close Panel on Exit?"=w329:bool)
            n107 = Select(t="UI: Front Panel State >> Close", s=w329, f="") -> (s? t:f=w326:string)
            n108 = call <vilib>:"Add State(s) to Queue__jki_lib_state_machine.vi"("State(s) in Front (\"\")"="Data: Cleanup\nEvents: Unregister\nProcess: Self Terminate", "State(s) in (\"\")"="Process: Sync", "State(s) at Back (\"\")"="Exit") -> ("States Out"=w321:string)  [unwired: 12 in]
            n109 = call <vilib>:"Add State(s) to Queue__jki_lib_state_machine.vi"("State(s) in Front (\"\")"="Macro: Write UI Config", "State(s) in (\"\")"=w326, "State(s) at Back (\"\")"=w321) -> ("States Out"=w325:string)  [unwired: 12 in]
            n110 = call <vilib>:"Add State(s) to Queue__jki_lib_state_machine.vi"("State(s) in Front (\"\")"=w325, "State(s) in (\"\")"=w332) -> ("States Out"=w331:string)  [unwired: 13 in]
          }
          frame "---------- Process ----------" {
            # "Template Separator\n(You can make a copy of, or modify, this frame)"
            n111 = call <vilib>:"Add State(s) to Queue__jki_lib_state_machine.vi"("State(s) in (\"\")"=w337) -> ("States Out"=w336:string)  [unwired: 14 in]
          }
          frame "Process: Sync" {
            n112 = Unbundle By Name(w345) -> ("Instrument UI"=w341:refnum<class "Instrument UI.Temperhum.lvclass">)
            n113 = call <vilib>:"WaitOnProcessSync.vi"("error in (no error)"=w340, "SMO"=w341) -> ("error out"=w339:errorcluster, "Don't run?"=w344:bool)  [unwired: 7 in, 1 out]
            n114 = Select(t="Data: Cleanup\nEvents: Unregister\nExit", s=w344, f="") -> (s? t:f=w338:string)
            n115 = call <vilib>:"Add State(s) to Queue__jki_lib_state_machine.vi"("State(s) in Front (\"\")"=w338, "State(s) in (\"\")"=w348) -> ("States Out"=w347:string)  [unwired: 13 in]
          }
          frame "Process: Self Terminate" {
            n116 = Unbundle By Name(w350) -> ("Instrument UI"=w349:refnum<class "Instrument UI.Temperhum.lvclass">)
            n117 = call <vilib>:"SelfTerminate.vi"("error in (no error)"=w352, "SMO in"=w349) -> ("error out"=w351:errorcluster)  [unwired: 8 in, 1 out]
            n118 = call <vilib>:"Add State(s) to Queue__jki_lib_state_machine.vi"("State(s) in (\"\")"=w355) -> ("States Out"=w354:string)  [unwired: 14 in]
          }
          frame "---------- Events ----------" {
            # "Template Separator\n(You can make a copy of, or modify, this frame)"
            n119 = call <vilib>:"Add State(s) to Queue__jki_lib_state_machine.vi"("State(s) in (\"\")"=w360) -> ("States Out"=w359:string)  [unwired: 14 in]
          }
          frame "Events: Register" {
            # "Expand to add\nmore events"
            # "Base Class Protected Events"
            n120 = Unbundle By Name(w374) -> ("Instrument UI"=w365:refnum<class "Instrument UI.Temperhum.lvclass">, "Instrument"=w364:refnum<class "Instrument.Temperhum.lvclass">)
            n121 = call <vilib>:"GetProtectedEvents.vi"("SMO"=w365) -> ("error out"=w368:errorcluster, "SMO Protected Events"=w372:T10)  [unwired: 8 in, 1 out]
            n122 = call <userlib>:"Instrument.GetPublicEvents.vi"("Instrument"=w364) -> ("error out"=w366:errorcluster, "Instrument Public Events"=w367:T11, "Instrument out"=w363:refnum<class "Instrument.Temperhum.lvclass">)  [unwired: 8 in]
            n123 = call "Instrument.Temperhum.GetPublicEvents.vi"("Instrument.Temperhum in"=w363) -> ("error out"=w362:errorcluster, "Temperhum Public Events"=w361:T12)  [unwired: 8 in, 1 out]
            n124 = register-events(w372, w367, w361) -> (reference out=w373:refnum<event-registration>, error out=w370:errorcluster)  [unwired: 2 in]
            n125 = Merge Errors(w362, w366, w371, w370, w368) -> (w369:errorcluster)
            n126 = call <vilib>:"Add State(s) to Queue__jki_lib_state_machine.vi"("State(s) in (\"\")"=w376) -> ("States Out"=w375:string)  [unwired: 14 in]
          }
          frame "Events: Unregister" {
            n127 = Unregister For Events(event registration refnum=w379, error in=w378) -> (error out=w377:errorcluster)
            n128 = call <vilib>:"Add State(s) to Queue__jki_lib_state_machine.vi"("State(s) in (\"\")"=w382) -> ("States Out"=w381:string)  [unwired: 14 in]
          }
          frame "---------- Configuration ----------" {
            # "Do not put any code in this frame.\n(It is a separator no-op. You can make a copy of this frame to create a new UI frame)"
            n129 = call <vilib>:"Add State(s) to Queue__jki_lib_state_machine.vi"("State(s) in (\"\")"=w387) -> ("States Out"=w386:string)  [unwired: 14 in]
          }
          frame "Configuration: Initialize" {
            # "Do not put any code in this frame.\n(It is a separator no-op. You can make a copy of this frame to create a new UI frame)"
            n130 = Unbundle By Name(w390) -> ("Configuration"=w388:refnum<class "Configuration.lvclass">, "Instrument"=w389:refnum<class "Instrument.Temperhum.lvclass">)
            n131 = call <vilib>:"GetName.vi"("error in (no error)"=w392, "SMO"=w389) -> ("error out"=w391:errorcluster, "Name"=w393:string)  [unwired: 6 in, 2 out]
            n132 = call <userlib>:"Default Path.vi"("error in (no error)"=w391, "Folder Name [Application Name]"=w393, "Configuration in"=w388) -> ("error out"=w394:errorcluster, "Configuration out"=w395:refnum<class "Configuration.lvclass">)  [unwired: 7 in]
            n133 = Bundle By Name(cluster=w390, "Configuration"=w395) -> (w396:T7)
            n134 = call <vilib>:"Add State(s) to Queue__jki_lib_state_machine.vi"("State(s) in (\"\")"=w399) -> ("States Out"=w398:string)  [unwired: 14 in]
          }
          frame "Configuration: Write UI Config File" {
            # "Do not put any code in this frame.\n(It is a separator no-op. You can make a copy of this frame to create a new Data frame)"
            n135 = Unbundle By Name(w404) -> ("Configuration"=w401:refnum<class "Configuration.lvclass">, "UI Cluster"=w403:T6)
            n136 = call <userlib>:"Write Configuration.vi"("error in (no error)"=w400, "Variant"=w403, "Configuration in"=w401) -> ("error out"=w402:errorcluster)  [unwired: 7 in, 1 out]
            n137 = call <vilib>:"Add State(s) to Queue__jki_lib_state_machine.vi"("State(s) in (\"\")"=w407) -> ("States Out"=w406:string)  [unwired: 14 in]
          }
          frame "Configuration: Read UI Config File" {
            # "Do not put any code in this frame.\n(It is a separator no-op. You can make a copy of this frame to create a new UI frame)"
            n138 = Unbundle By Name(w410) -> ("UI Cluster"=w413:T6, "Configuration"=w416:refnum<class "Configuration.lvclass">)
            n139 = call <userlib>:"Read Configuration.vi"("INI Fomatted Cluster Type"=w413, "error in (no error)"=w412, "Configuration in"=w416) -> ("error out"=w415:errorcluster, "Configuration"=w414:variant)  [unwired: 6 in, 1 out]
            n140 = Variant To Data(error in=w415, type=w413, Variant=w414) -> (data=w409:T6, error out=w411:errorcluster)
            n141 = Bundle By Name(cluster=w410, "UI Cluster"=w409) -> (w408:T7)
            n142 = call <vilib>:"Add State(s) to Queue__jki_lib_state_machine.vi"("State(s) in (\"\")"=w419) -> ("States Out"=w418:string)  [unwired: 14 in]
          }
          frame "---------- Action ----------" {
            n143 = Unbundle By Name(w422) -> ("Instrument UI"=w420:refnum<class "Instrument UI.Temperhum.lvclass">)
            n144 = Bundle By Name(cluster=w422, "Instrument UI"=w420) -> (w421:T7)
            n145 = call <vilib>:"Add State(s) to Queue__jki_lib_state_machine.vi"("State(s) in (\"\")"=w426) -> ("States Out"=w425:string)  [unwired: 14 in]
          }
          frame "Action: Notify UI Closed" {
            # "Notify that the UI has been closed"
            n146 = Unbundle By Name(w427) -> ("Instrument UI"=w430:refnum<class "Instrument UI.Temperhum.lvclass">)
            n147 = call <vilib>:"Hide.vi"("error in (no error)"=w429, "SMO.UI"=w430) -> ("error out"=w428:errorcluster)  [unwired: 8 in, 1 out]
            n148 = call <vilib>:"Add State(s) to Queue__jki_lib_state_machine.vi"("State(s) in (\"\")"=w433) -> ("States Out"=w432:string)  [unwired: 14 in]
          }
          frame "Action: getAll" {
            n149 = Unbundle By Name(w437) -> ("getAll"=w435:T4, "Instrument"=w440:refnum<class "Instrument.Temperhum.lvclass">)
            n150 = call "GET ALL.vim"("type"=w435, "error in (no error)"=w438, "Instrument in"=w440) -> ("error out"=w442:errorcluster, "getAll"=w434:T4, "Instrument out"=w436:refnum<class "Instrument.Temperhum.lvclass">)  [unwired: 6 in]
            n151 = Bundle By Name(cluster=w437, "Instrument"=w436, "getAll"=w434) -> (w439:T7)
            n152 = call <vilib>:"Add State(s) to Queue__jki_lib_state_machine.vi"("State(s) in Front (\"\")"="" ("State(s) in Front (\"\")"), "State(s) in (\"\")"=w445) -> ("States Out"=w444:string)  [unwired: 13 in]
          }
          frame "Action: setConfiguration" {
            n153 = Unbundle By Name(w448) -> ("Instrument"=w451:refnum<class "Instrument.Temperhum.lvclass">, "Config Cluster"=w446:T5)
            n154 = call "SET CONFIG.vim"("error in (no error)"=w449, "Configuration"=w446, "Instrument in"=w451) -> ("error out"=w453:errorcluster, "Instrument out"=w447:refnum<class "Instrument.Temperhum.lvclass">)  [unwired: 7 in]
            n155 = Bundle By Name(cluster=w448, "Instrument"=w447) -> (w450:T7)
            n156 = call <vilib>:"Add State(s) to Queue__jki_lib_state_machine.vi"("State(s) in Front (\"\")"="" ("State(s) in Front (\"\")"), "State(s) in (\"\")"=w456) -> ("States Out"=w455:string)  [unwired: 13 in]
          }
        }
      }
    }
    frame Error {
    }
  }
  n157 = call-parent "Process.vi"("error in"=w8, "Instrument UI in"=w7) -> ("error out"=w5:errorcluster, "Instrument UI out"=→"Instrument UI.FrameworkTemplate out":refnum<class "Instrument UI.Temperhum.lvclass">)  [unwired: 8 in]
  n158 = Merge Errors(w5, w4) -> (→"error out":errorcluster)
